vi "MFC write REG.vi"(10 "UnitID":string="A", 11 "VISA resource name":refnum<visa-resource-name>="COM1") -> (0 "error out":errorcluster={"status"=FALSE, "code"=0, "source"="VISA Read in ReadSerialBuffer.vi->AlicatSetPoint.vi->AlicatWrite8V2.vi"}, 1 "AlicatResponse":string="A +013.53 +023.20 +0000.0 +0000.0 0250.0     Air\r")   [LabVIEW 2011]
uses:
  <vilib>/Instr/_visa.llb/VISA Configure Serial Port (Instr).vi
panel:
  in  "RegisterValue":i32=18375
  in  "RegisterNum":i16=16 min=0 max=79 step=1
  # "18375 only mass"
  # "199 normal"
  # "0= 0%\n64000 = 100%"
  # "Read this response from the change the setpoint write.\nClears the Serial in buffer"
  # "Code 1073676294 is\nokay since we are only\nreading one byte till we\nget to the end of message\nbyte."
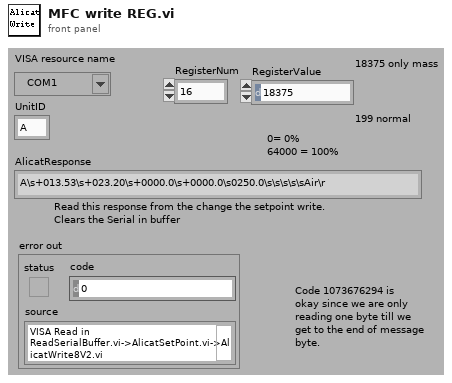
[diagram p1: front panel]
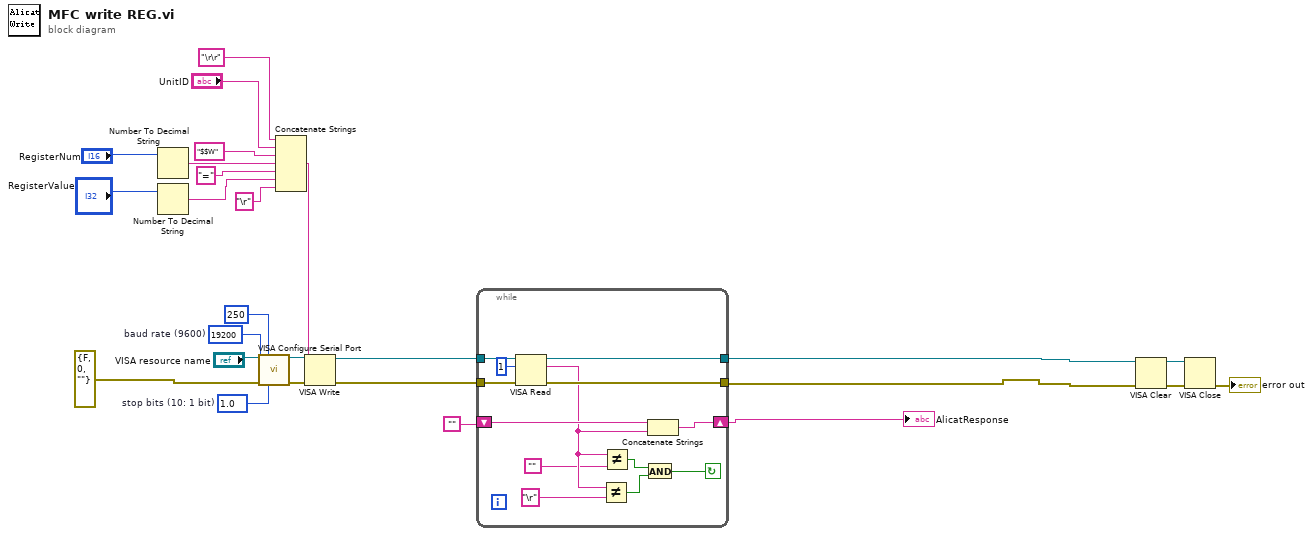
[diagram p0: block diagram]
diagram:
  w24 = u16 10 items=["1.0"=10, "1.5"=15, "2.0"=20]  # stop bits (10: 1 bit)
  w25 = u32 19200  # baud rate (9600)
  n1 = Number To Decimal String(number="RegisterNum") -> (decimal integer string=w4:string)  [unwired: 1 in]
  n2 = Number To Decimal String(number="RegisterValue") -> (decimal integer string=w2:string)  [unwired: 1 in]
  n3 = call-poly "VISA Configure Serial Port"("VISA resource name"="VISA resource name", "timeout (10sec)"=u32 250, "baud rate (9600)"=w25, "error in (no error)"=errorcluster {"status"=FALSE, "code"=0, "source"=""}, "stop bits (10: 1 bit)"=w24) -> ("VISA resource name out"=w21:refnum<visa-resource-name>, "error out"=w20:errorcluster)  [unwired: 9 in]
  n4 = Concatenate Strings("\r\r" ("string"), "UnitID", "$$W" ("write buffer (\"\")"), w4, "=" ("string"), w2, "\r" ("string")) -> (w15:string)
  n5 = VISA Write(VISA resource name=w21, write buffer=w15, error in (no error)=w20) -> (VISA resource name out=w17:refnum<visa-resource-name>, error out=w16:errorcluster)  [unwired: 1 out]
  n6 = while {
    tunnel: [w38] -> w8
    tunnel: [w37] -> w9
    shift-right: [w35] -> w10
    shift-left: "" -> [w34]
    tunnel: w17 -> [w28]
    tunnel: w16 -> [w27]
    stop <- w30 continue-if-true
    n7 = VISA Read(VISA resource name=w28, byte count=u32 1 ("byte count (0)"), error in (no error)=w27) -> (VISA resource name out=w37:refnum<visa-resource-name>, read buffer=w33:string, error out=w38:errorcluster)  [unwired: 1 out]
    n8 = Not Equal?(x=w33, y="\r") -> (x != y?=w31:bool)
    n9 = Not Equal?(x=w33, y="") -> (x != y?=w32:bool)
    n10 = And(x=w32, y=w31) -> (x .and. y?=w30:bool)
    n11 = Concatenate Strings(w34, w33) -> (w35:string)
  }
  "AlicatResponse" <- w10
  n12 = VISA Clear(VISA resource name=w9, error in (no error)=w8) -> (VISA resource name out=w19:refnum<visa-resource-name>, error out=w18:errorcluster)
  n13 = VISA Close(VISA resource name=w19, error in (no error)=w18) -> (error out=→"error out":errorcluster)
